vi "To File (Ref).vi"(6 "enable LabVIEW extensions? (T)":bool=TRUE, 7 "Pretty Print?":bool=TRUE, 8 "error in (no error)":errorcluster, 10 "Variant in":variant, 11 "refnum in":refnum<file>) -> (0 "error out":errorcluster, 3 "refnum out":refnum<file>)   [LabVIEW 2020, in "Variant JSON API.lvlib"]
doc: "Saves a JSON instance's data to the given file."
uses:
  Variant JSON API.lvlib
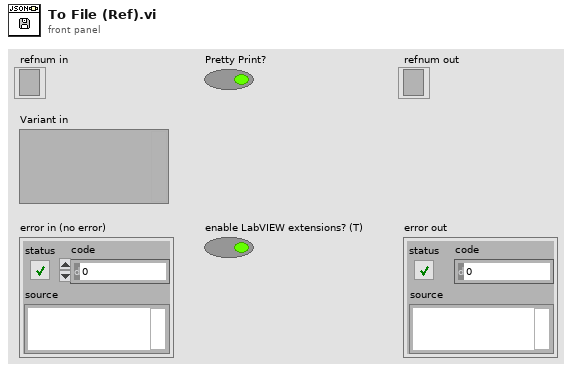
[diagram p1: front panel]
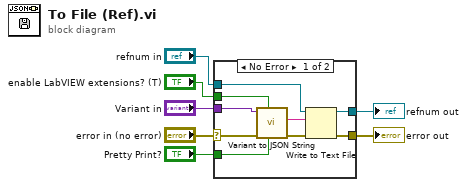
[diagram p0: block diagram]
diagram:
  n1 = case shown="No Error" "error in (no error)" {
    selector: "error in (no error)" -> [w15 w18]
    tunnel: "Variant in" -> [w16 _]
    tunnel: [w12 w18] -> w5
    tunnel: "Pretty Print?" -> [w10 _]
    tunnel: "refnum in" -> [w13 w17]
    tunnel: [w11 w17] -> w2
    tunnel: "enable LabVIEW extensions? (T)" -> [w9 _]
    frame No Error {
      n2 = call "Variant to JSON String.vi"("enable LabVIEW extensions? (T)"=w9, "pretty print? (F)"=w10, "error in (no error)"=w15, "Variant in"=w16) -> ("error out"=w14:errorcluster, "String"=w8:string)  [unwired: 5 in, 1 out]
      n3 = Write to Text File(file (use dialog)=w13, text=w8, error in=w14) -> (refnum out=w11:refnum<file>, error out=w12:errorcluster)  [unwired: 1 in, 1 out]
    }
    frame Error {
    }
  }
  "error out" <- w5
  "refnum out" <- w2
